vi "SICK Init.vi"(7 "SICK Init Timeout":i32=2000, 8 "error in":errorcluster, 10 "SICK Commands":string[][](array[string]), 11 "FPGA_MAIN ref in":T1) -> (0 "error out":errorcluster, 2 "Init Success":bool, 3 "FPGA_MAIN ref out":T1)   [LabVIEW 2009]
uses:
  TypeDefs/Sensor TypeDefs/FPGA Main ref.ctl
  <vilib>/rvi/interface/nirviReadWriteControl/nirviReadWriteControl.xnode
  FPGA Bitfiles/Q_IGVC_2010.lvproj_FPGA Target_FPGA_MAIN.vi.lvbitx
  <vilib>/Utility/error.llb/Error Cluster From Error Code.vi
  <vilib>/rvi/errors/niLvFpgaAdjustHostInterfaceError.vi
  <vilib>/rvi/interface/common/niFpgaNodeNameForErrorReporting.ctl
  <vilib>/rvi/errors/niLvFpgaWhatHappensToTopLevelVI.ctl
  <vilib>/rvi/interface/nirviMethod/nirviMethod.xnode
  <vilib>/LabVIEW Targets/FPGA/RIO/nirio_HostInterface/nirio_WaitOnIRQ.vi
  <vilib>/RVI Host/nirviSupport.llb/nirviErrorClusterFromErrorCode.vi
  NiRioSrv.dll
panel:
  out "Correct Response Read?":bool
  out "Initialization success":bool
  out "Commands":u8[](array[numeric])=[8, 2, 0, 2, 0, 32, 36, 52, 8, 0, 0, 0, 0, 0, 0, 0, 0, 7, 6, 2, 128, 3, 0, 160, 0, 0, 0, 0, 0, 0, 0, 0] format="%x"
  out "Response":u8[](array[numeric])=[6, 2, 128, 3, 0, 160, 0] format="%x"
  out "Command":u8[](array[numeric])=[2, 0, 2, 0, 32, 36, 52, 8] format="%x"
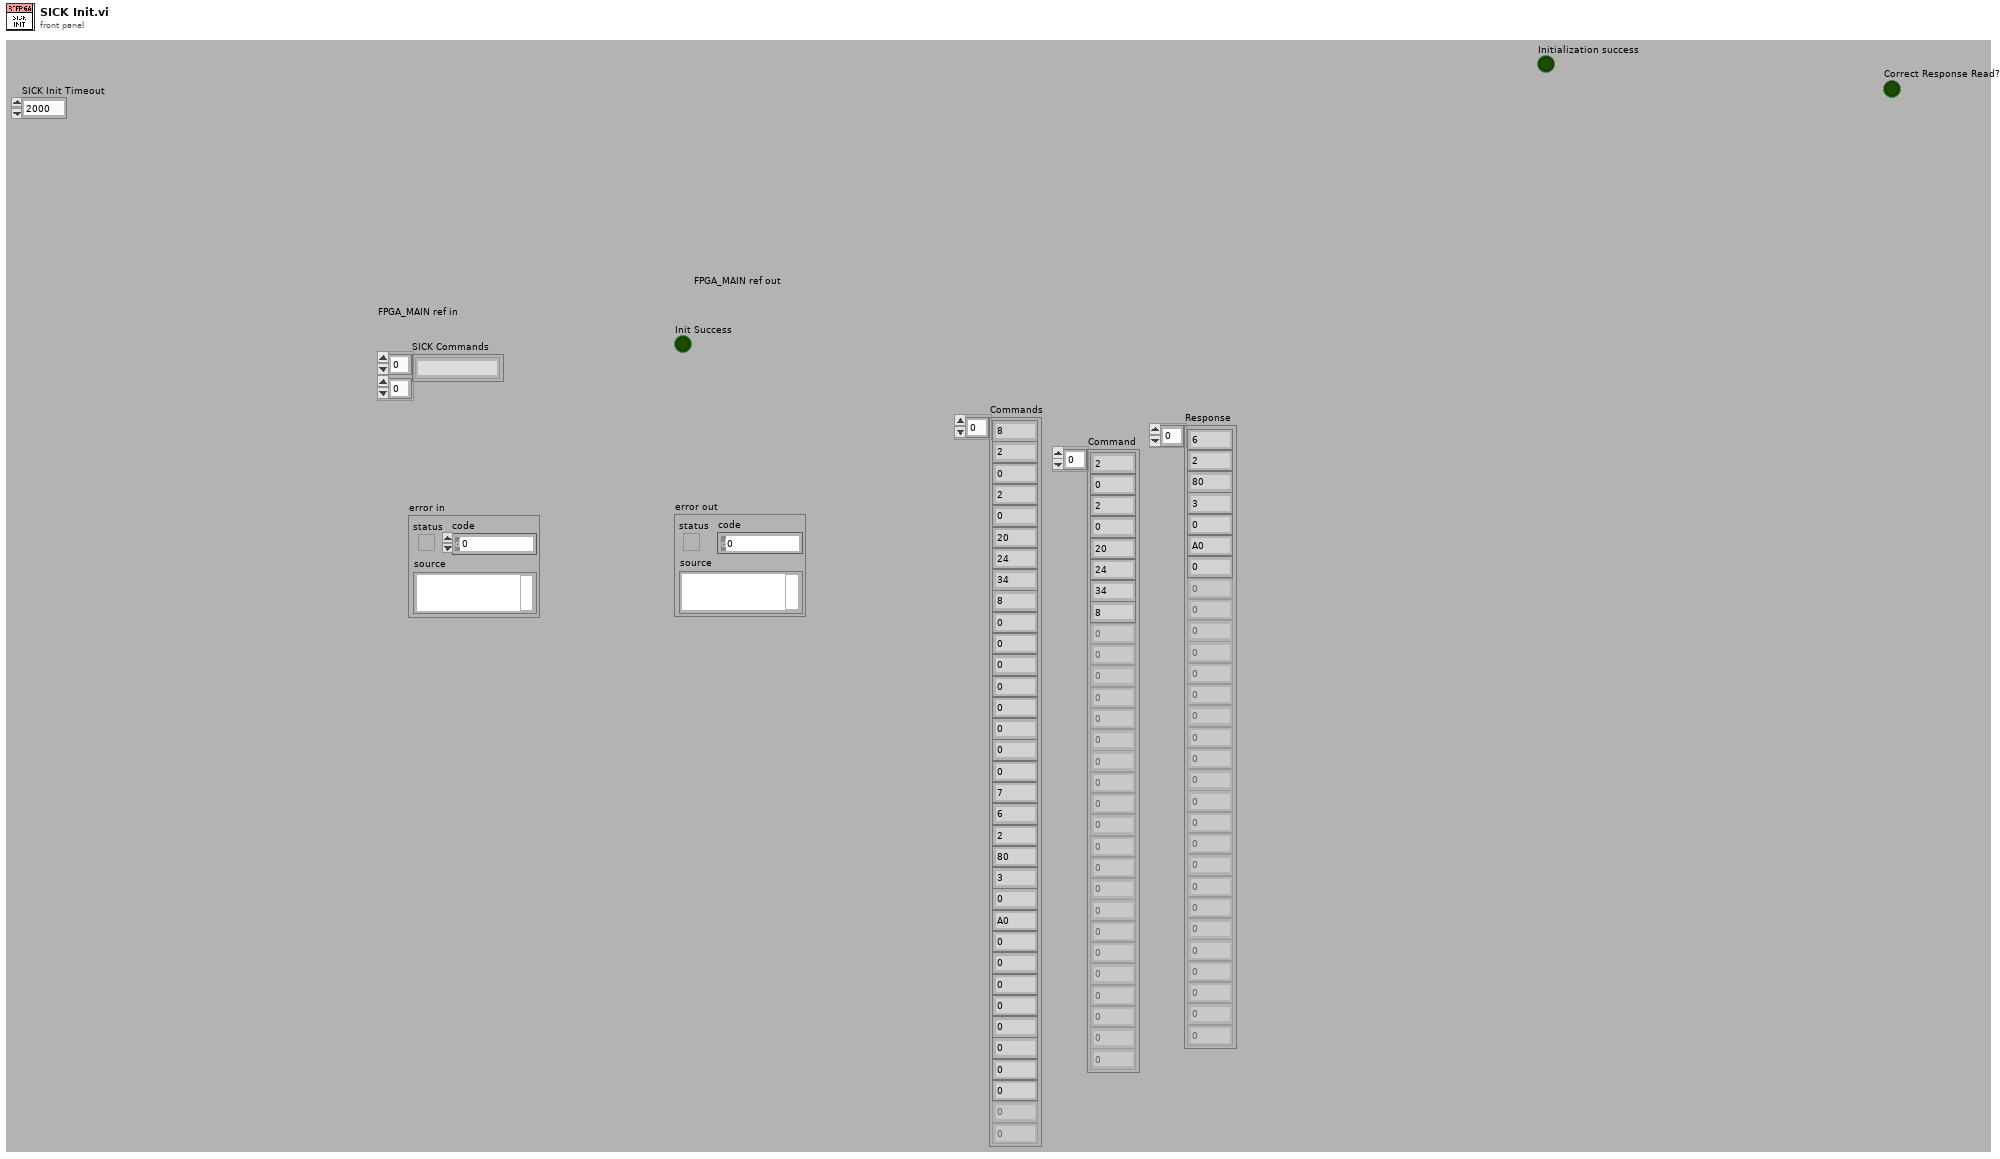
[diagram p1: front panel]
types:
  T1 = typedef "FPGA Main ref.ctl" = refnum<k20>
  T2 = typedef "niFpgaNodeNameForErrorReporting.ctl" = enum16{"Open FPGA VI Reference", "Read/Write Control", "Invoke Method: Abort", "Invoke Method: Acknowledge IRQ", "Invoke Method: Download", "Invoke Method: FIFO.Configure", "Invoke Method: FIFO.Read", "Invoke Method: FIFO.Start", "Invoke Method: FIFO.Stop", "Invoke Method: FIFO.Write", "Invoke Method: Reset", "Invoke Method: Run", "Invoke Method: Wait on IRQ", "Close FPGA VI Reference"}
  T3 = typedef "niLvFpgaWhatHappensToTopLevelVI.ctl" = enum16{"top level VI scripted behind XNode", "top level VI inlined behind XNode"}
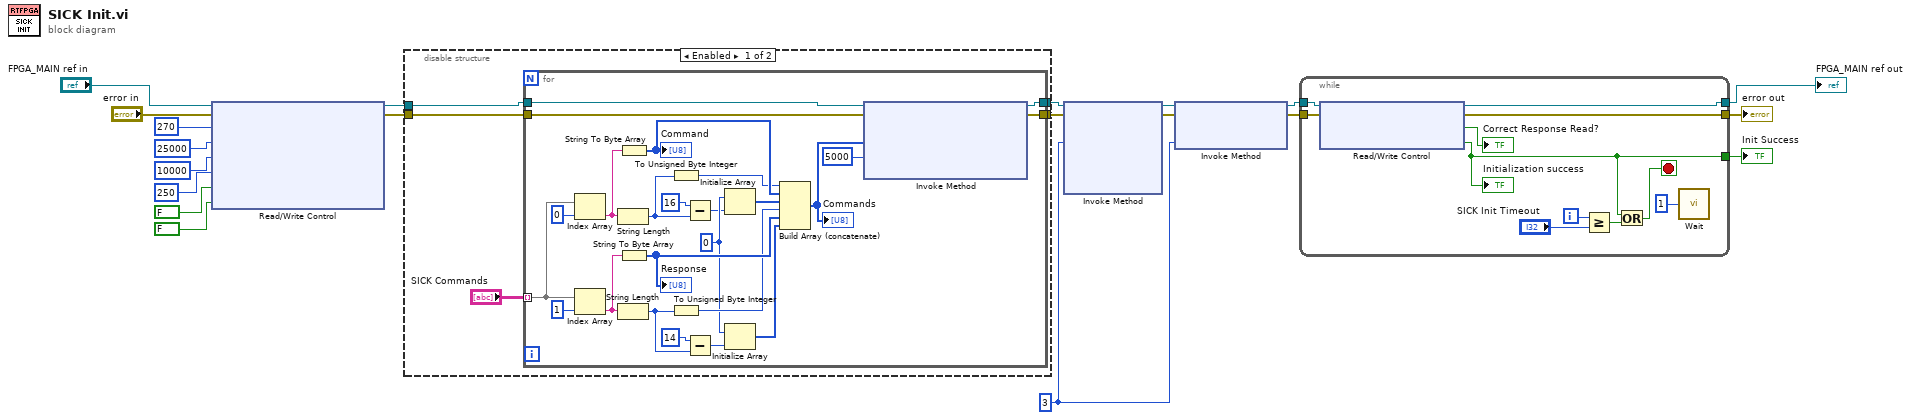
[diagram p0: block diagram]
diagram:
  w3 = 3 ("IRQ Number(s)")
  n1 = xnode "Read/Write Control"("FPGA VI Reference In"="FPGA_MAIN ref in", "error in"="error in", "Overflow Reading"=u16 270, "Bytes at Port Timeout (us)"=25000, "Set new baud rate wait (usec)"=u32 10000, "Read/Write Timeout (ms)"=250, "En overflow replacement"=FALSE, "EN mask overflow bytes"=FALSE) -> ("FPGA VI Reference Out"=w10:T1, "error out"=w9:errorcluster)
  n2 = disable-structure shown="Enabled" {
    disable-tunnel: w10 -> [w25 _]
    disable-tunnel: w9 -> [w24 _]
    disable-tunnel: [w23 _] -> w2
    disable-tunnel: [w22 _] -> w1
    frame #0 {
      n3 = for {
        tunnel: [w44] -> w23
        tunnel: [w43] -> w22
        tunnel: "SICK Commands" -> [w28] mode=indexing
        tunnel: w25 -> [w27]
        tunnel: w24 -> [w26]
        w37 = u8 0 ("index")
        n4 = Index Array(array=w28, index=0) -> (element=w47:string)
        n5 = Index Array(array=w28, index=1) -> (element=w45:string)
        n6 = String Length(string=w47) -> (length=w35:i32)
        n7 = String Length(string=w45) -> (length=w30:i32)
        n8 = String To Byte Array(string=w47) -> (unsigned byte array=w46:u8[])
        "Command" <- w46
        n9 = String To Byte Array(string=w45) -> (unsigned byte array=w41:u8[])
        "Response" <- w41
        n10 = To Unsigned Byte Integer(number=w35) -> (unsigned 8bit integer=w36:u8)
        n11 = To Unsigned Byte Integer(number=w30) -> (unsigned 8bit integer=w40:u8)
        n12 = Subtract(x=16 ("y"), y=w35) -> (x-y=w33:i32)
        n13 = Subtract(x=14 ("y"), y=w30) -> (x-y=w32:i32)
        n14 = Initialize Array(w37, w33) -> (w38:u8[])
        n15 = Initialize Array(w37, w32) -> (w39:u8[])
        n16 = Build Array (concatenate)(w36, w46, w38, w40, w41, w39) -> (w42:u8[])
        "Commands" <- w42
        n17 = xnode "Invoke Method"("FPGA VI Reference In"=w27, "error in"=w26, "Data"=w42, "Timeout (ms)"=5000) -> ("FPGA VI Reference Out"=w44:T1, "error out"=w43:errorcluster)  [unwired: 1 out]
      }
    }
    frame #1 {
    }
  }
  n18 = xnode "Invoke Method"("FPGA VI Reference In"=w2, "error in"=w1, "IRQ Number(s)"=w3) -> ("FPGA VI Reference Out"=w4:T1, "error out"=w5:errorcluster)  [unwired: 3 out]
  n19 = xnode "Invoke Method"("FPGA VI Reference In"=w4, "error in"=w5, "IRQ Number(s)"=w3) -> ("FPGA VI Reference Out"=w12:T1, "error out"=w11:errorcluster)
  n20 = while {
    tunnel: w12 -> [w126]
    tunnel: [w122] -> w7
    tunnel: w11 -> [w125]
    tunnel: [w124] -> w8
    tunnel: [w116] -> w6
    i -> [w120]
    stop <- w118 stop-if-true
    n21 = xnode "Read/Write Control"("FPGA VI Reference In"=w126, "error in"=w125) -> ("FPGA VI Reference Out"=w124:T1, "error out"=w122:errorcluster, "Correct Response Read?"=→"Correct Response Read?":bool, "Initialization success"=w116:bool)
    "Initialization success" <- w116
    n22 = Greater Or Equal?(x=w120, y="SICK Init Timeout") -> (x >= y?=w117:bool)
    n23 = Or(x=w116, y=w117) -> (x .or. y?=w118:bool)
    n24 = call "Wait"("Count(mSec)"=u32 1 ("milliseconds to wait")) -> ()  [unwired: 1 out]
  }
  "FPGA_MAIN ref out" <- w8
  "error out" <- w7
  "Init Success" <- w6
